vi "Constants.vi"() -> ()   [LabVIEW 2019, in "MD4Logger Shared.lvlib"]
doc: "Use this Global VI to access the GUIDs assigned to the page resources of the Custom Device."
uses:
  MD4Logger Shared.lvlib
panel:
  in  "Tab Control":enum32{"GUIDS", "Constants", "Properties"}(tab)
  in  "MD4Logger":string="1a3b2b0d-9cf3-4849-bac1-3a09abcb7558"
  in  "Channels Folder":string="2a3b2b0d-9cf3-4849-bac1-3a09abcb7558"
  in  "Folder Path":string="3a3b2b0d-9cf3-4849-bac1-3a09abcb7558"
  in  "Compiled.Settings":string="Compiled.Settings"
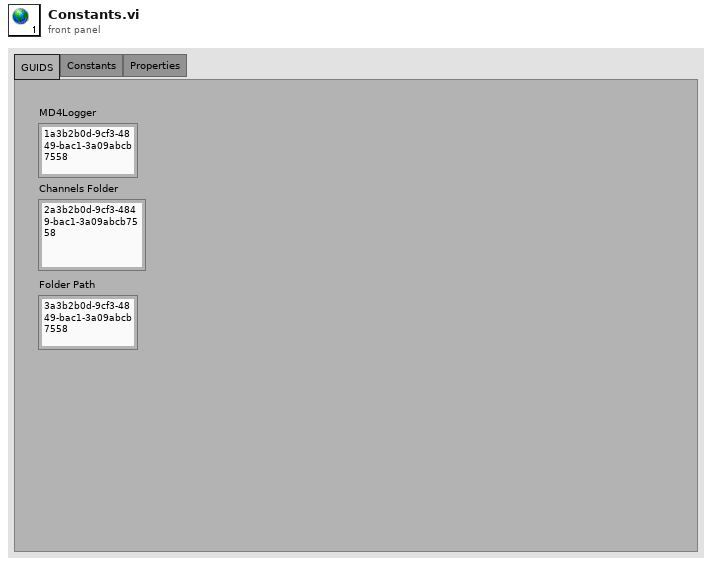
[diagram p1: front panel]
diagram:
